vi "Initialize.vi"(8 "error in (no error)":errorcluster, 11 "CT-Energize-Cmd in":refnum<class "CT-Energize-Cmd.lvclass">) -> (0 "error out":errorcluster, 3 "CT-Energize-Cmd out":refnum<class "CT-Energize-Cmd.lvclass">)   [LabVIEW 2013, in "CT-Energize-Cmd.lvclass"]
uses:
  CT-Energize-Cmd.lvclass
  States/CT-Energizing-State/CT-Energizing-State.lvclass
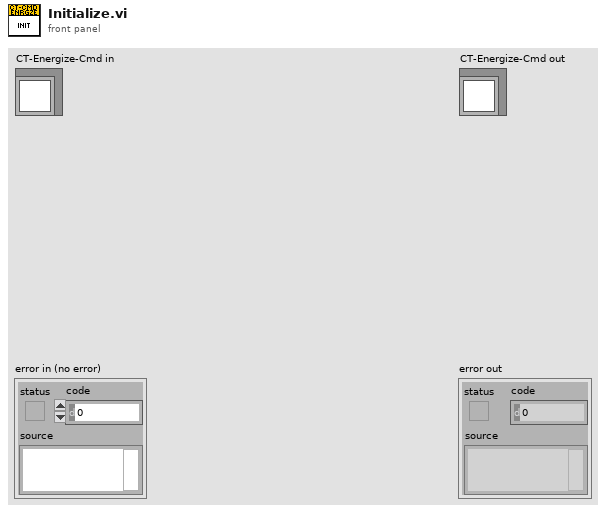
[diagram p1: front panel]
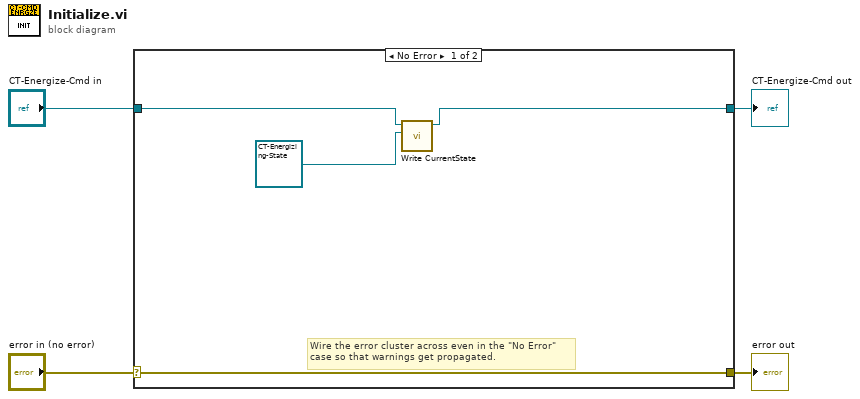
[diagram p0: block diagram]
diagram:
  n1 = case shown="No Error" "error in (no error)" {
    selector: "error in (no error)" -> [w8 w10]
    tunnel: [w8 w10] -> w3
    tunnel: [w6 w9] -> w1
    tunnel: "CT-Energize-Cmd in" -> [w7 w9]
    frame No Error {
      # "Wire the error cluster across even in the \"No Error\"\ncase so that warnings get propagated."
      n2 = call-dynamic "Write CurrentState.vi"("State.lvclass"=refnum<class "CT-Energizing-State.lvclass"> refnum ("CT-Energizing-State.lvclass"), "Command in"=w7) -> ("Command out"=w6:refnum<class "CT-Energize-Cmd.lvclass">)  [unwired: 8 in, 1 out]
    }
    frame Error {
    }
  }
  "error out" <- w3
  "CT-Energize-Cmd out" <- w1
